vi "Calculate Register X.vi"(1 "Instructions":string[](array[string])) -> (0 "Register X":map{i32, i32}(c390))   [LabVIEW 2020, in "AoC 2022.lvlib"]
uses:
  AoC 2022.lvlib
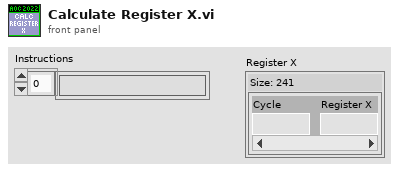
[diagram p1: front panel]
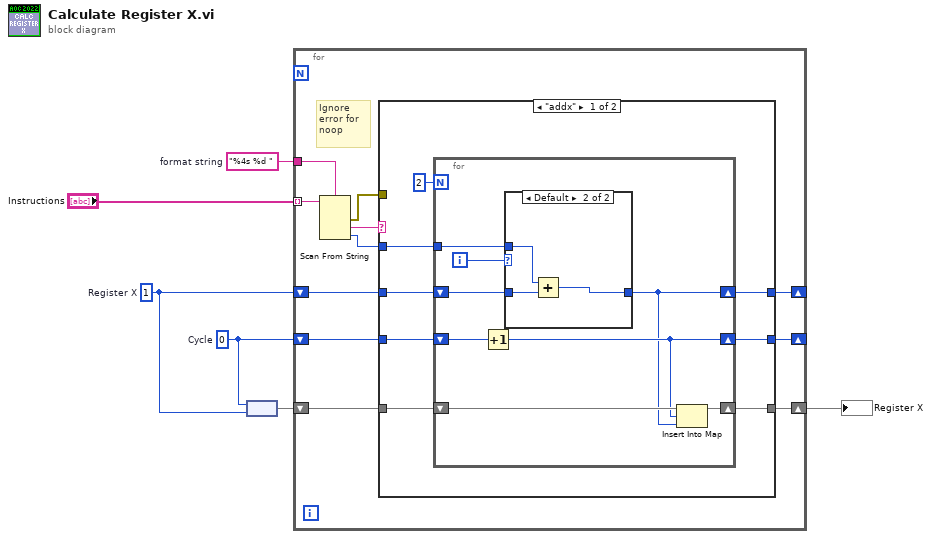
[diagram p0: block diagram]
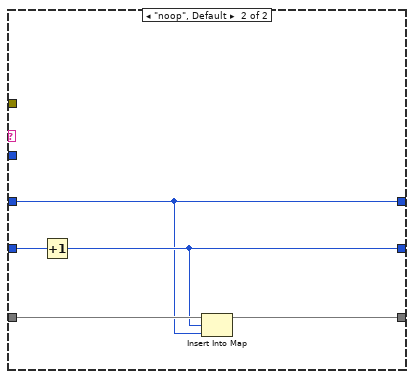
[diagram p3: hidden frame]
diagram:
  w4 = 1  # Register X
  w6 = 0  # Cycle
  w2 = "%4s %d "  # format string
  n1 = node(w6, w4) -> (w5:map{i32, i32})
  n2 = for {
    tunnel: "Instructions" -> [w17] mode=indexing
    tunnel: w2 -> [w16]
    shift-right: [w12] -> _
    shift-left: w6 -> [w13]
    shift-right: [w8] -> w3
    shift-left: w5 -> [w11]
    shift-right: [w9] -> _
    shift-left: w4 -> [w10]
    # "Ignore error for noop"
    n3 = Scan From String(format string=w16, input string=w17) -> (error out=w7:errorcluster, output 1=w15:string, output 2=w14:i32)  [unwired: 4 in, 2 out]
    n4 = case shown="\"addx\"" w15 {
      tunnel: w14 -> [w18 _]
      tunnel: w13 -> [w24 w42]
      tunnel: [w23 w39] -> w12
      tunnel: w11 -> [w21 w41]
      tunnel: w10 -> [w22 w38]
      tunnel: [w19 w38] -> w9
      tunnel: [w20 w40] -> w8
      tunnel: w7 -> [_ _]
      frame "addx" {
        n5 = for {
          N: 2 -> [_]
          shift-right: [w27] -> w23
          shift-left: w24 -> [w33]
          shift-right: [w30] -> w20
          shift-left: w21 -> [w31]
          shift-right: [w26] -> w19
          shift-left: w22 -> [w32]
          tunnel: w18 -> [w28]
          i -> [w29]
          n6 = Increment(x=w33) -> (x+1=w27:i32)
          n7 = case shown="Default" w29 {
            tunnel: w32 -> [w34 w36]
            tunnel: [w34 w35] -> w26
            tunnel: w28 -> [_ w37]
            frame 0 {
            }
            frame Default {
              n8 = Add(x=w37, y=w36) -> (x+y=w35:i32)
            }
          }
          n9 = Insert Into Map(map in=w31, key=w27, value=w26) -> (map out=w30:map{i32, i32})  [unwired: 2 out]
        }
      }
      frame "noop", Default {
        n10 = Increment(x=w42) -> (x+1=w39:i32)
        n11 = Insert Into Map(map in=w41, key=w39, value=w38) -> (map out=w40:map{i32, i32})  [unwired: 2 out]
      }
    }
  }
  "Register X" <- w3
